vi "Service_Setup.vi"(0 "Log in":T3[](array[typedef]), 1 "ROS":T1={"topic port"=1236, "Node"="/labview", "topic"="/robot/head/command_head_nod", "type"="std_msgs/Bool", "node port"=7000, "error "={"status"=FALSE, "code"=0, "source"=""}, "Direction"=enum."Publisher", "APIs"=[], "Update (ms)"=1, "write queue"=1}, 2 "Msg to Send":string, 3 "Subscriber":T4) -> (5 "Log out":T3[](array[typedef]), 6 "Reply":string, 7 "error out":errorcluster)   [LabVIEW 2012]
doc: "Creates and sends the connection header and message to a service provider. Implemented in the background server."
uses:
  <userlib>/rosforlv/ROS/Code/Console/Servers/ServerSubs/ROSLog.ctl
  <userlib>/rosforlv/ROS/Code/SubVIs/_ROSControl.ctl
  <userlib>/rosforlv/ROS/Code/SubVIs/_ROSDirection.ctl
  <userlib>/rosforlv/ROS/Code/_ROSDefinition.vi
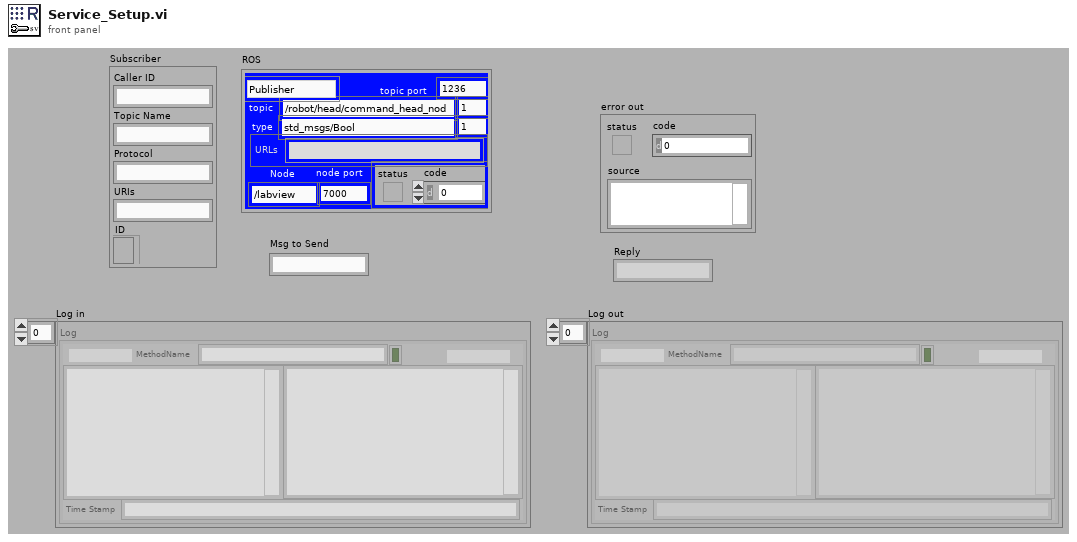
[diagram p1: front panel]
types:
  T1 = typedef "_ROSControl.ctl" = cluster{"topic port":u16, "Node":string, "topic":string, "type":string, "node port":u32, "error ":errorcluster, "Direction":T2, "APIs":string[], "Update (ms)":u16, "write queue":u16}
  T2 = typedef "_ROSDirection.ctl" = enum16{"Node", "Publisher", "Subscriber", "Service Client"}
  T3 = typedef "ROSLog.ctl" = cluster{"Sent":string, "Reply":string, "MethodName":string, "success":bool, "Dir1":string, "Dir2":string, "Time Stamp":string}
  T4 = cluster{"Caller ID":string, "Topic Name":string, "Protocol":string, "URIs":string, "ID":refnum<k5>}
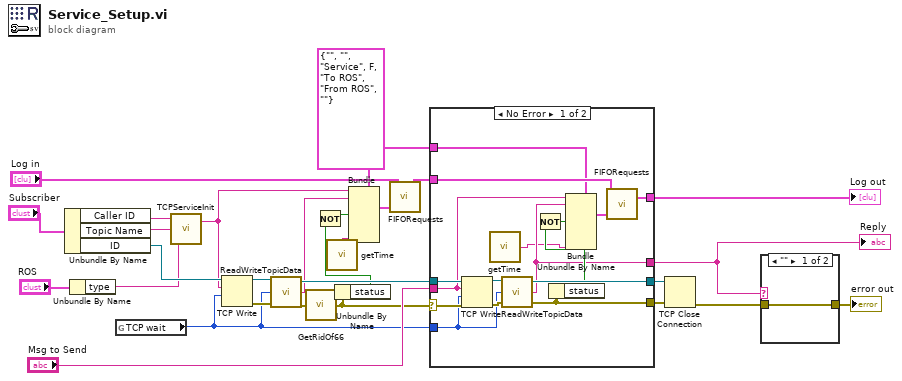
[diagram p0: block diagram]
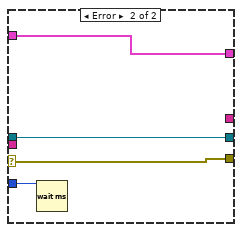
[diagram p2: hidden frame]
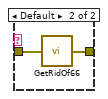
[diagram p3: hidden frame]
diagram:
  w5 = T3 {"Sent"="", "Reply"="", "MethodName"="Service", "success"=FALSE, "Dir1"="To ROS", "Dir2"="From ROS", "Time Stamp"=""} ("Log")
  n1 = Unbundle By Name("Subscriber") -> ("Caller ID"=w27:string, "Topic Name"=w26:string, "ID"=w19:refnum<k5>)
  n2 = Unbundle By Name("ROS") -> ("type"=w2:string)
  n3 = global read "_ROSDefinition.vi" "TCP wait"() -> (w1:i32)
  n4 = call <userlib>:"TCPServiceInit.vi"("Type"=w2, "topic"=w26, "callerID"=w27) -> ("TCP ROS Reply"=w15:string)  [unwired: 1 out]
  n5 = TCP Write(connection ID=w19, data in=w15, 9:w1) -> (connection ID out=w18:refnum<k5>, error out=w17:errorcluster)  [unwired: 1 in, 1 out]
  n6 = call <userlib>:"ReadWriteTopicData.vi"("error in (no error)"=w17, "timeout ms (1000)"=w1, "connection ID in"=w18) -> ("error out"=w8:errorcluster, "data out"=w4:string, "connection ID out"=w16:refnum<k5>)
  n7 = call <userlib>:"GetRidOf66.vi"("error in (no error)"=w8) -> ("error out"=w7:errorcluster)
  n8 = call <userlib>:"getTime.vi"() -> ("Current Time"=w6:string)  [unwired: 1 in]
  n9 = Unbundle By Name(w7) -> ("status"=w12:bool)
  n10 = Not(x=w12) -> (.not. x?=w11:bool)
  n11 = Bundle(cluster=w5, "Sent"=w15, "Reply"=w4, "success"=w11, "Time Stamp"=w6) -> (w14:T3)  [unwired: 3 in]
  n12 = call <userlib>:"FIFORequests.vi"("Log"=w14, "Requests in"="Log in") -> ("Requests out"=w9:T3[])  [unwired: 1 in]
  n13 = case shown="No Error" w7 {
    selector: w7 -> [w40 w46]
    tunnel: w16 -> [w42 w47]
    tunnel: w1 -> [w31 w48]
    tunnel: [w41 w47] -> w13
    tunnel: [w36 w46] -> w10
    tunnel: w9 -> [w38 w45]
    tunnel: [w37 w45] -> w24
    tunnel: "Msg to Send" -> [w32 _]
    tunnel: [w33 _] -> w22
    tunnel: w5 -> [w29 _]
    frame No Error {
      n14 = TCP Write(connection ID=w42, data in=w32, error in (no error)=w40, 9:w31) -> (connection ID out=w44:refnum<k5>, error out=w43:errorcluster)  [unwired: 1 out]
      n15 = call <userlib>:"getTime.vi"() -> ("Current Time"=w30:string)  [unwired: 1 in]
      n16 = call <userlib>:"ReadWriteTopicData.vi"("error in (no error)"=w43, "timeout ms (1000)"=w31, "connection ID in"=w44) -> ("error out"=w36:errorcluster, "data out"=w33:string, "connection ID out"=w41:refnum<k5>)
      n17 = Unbundle By Name(w36) -> ("status"=w35:bool)
      n18 = Not(x=w35) -> (.not. x?=w34:bool)
      n19 = Bundle(cluster=w29, "Sent"=w32, "Reply"=w33, "success"=w34, "Time Stamp"=w30) -> (w39:T3)  [unwired: 3 in]
      n20 = call <userlib>:"FIFORequests.vi"("Log"=w39, "Requests in"=w38) -> ("Requests out"=w37:T3[])  [unwired: 1 in]
    }
    frame Error {
      n21 = Wait (ms)(milliseconds to wait=w48) -> ()  [unwired: 1 out]
    }
  }
  "Log out" <- w24
  "Reply" <- w22
  n22 = TCP Close Connection(connection ID=w13, error in (no error)=w10) -> (error out=w21:errorcluster)  [unwired: 1 in, 1 out]
  n23 = case shown="\"\"" w22 {
    tunnel: w21 -> [w49 w51]
    tunnel: [w49 w50] -> w20
    frame "" {
    }
    frame Default {
      n24 = call <userlib>:"GetRidOf66.vi"("error in (no error)"=w51) -> ("error out"=w50:errorcluster)
    }
  }
  "error out" <- w20
